vi "Charact One Point.vi"(0 "SG Path in":refnum<class "SG 18GHz Path.lvclass">, 5 "Cal point in":T1, 11 "error in (no error)":errorcluster) -> (4 "SG Path out":refnum<class "SG 18GHz Path.lvclass">, 15 "error out":errorcluster)   [LabVIEW 2023, in "RFFixtureCharact.RFPM.lvlib" / "SG 18GHz Path.lvclass"]
uses:
  SG 18GHz Path.lvclass
  Public/Base Classes/Scalar/Scalar Path/Type Definitions/Cal Point.ctl
  Public/Base Classes/Scalar/SG Abstract Path/SG Abstract Path.lvclass
  Public/Base Classes/Scalar/Scalar Path/Scalar Path.lvclass
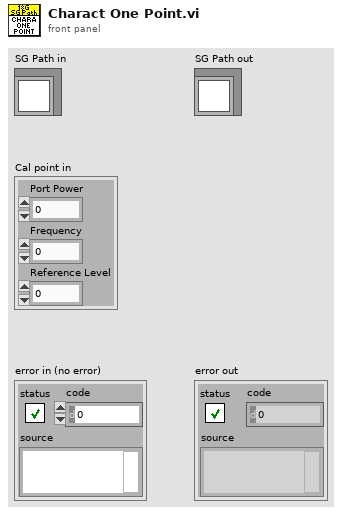
[diagram p1: front panel]
types:
  T1 = typedef "RFFixtureCharact.Public.lvlib/Scalar Path.lvclass/Cal Point.ctl" = cluster{"Port Power":dbl, "Frequency":dbl, "Reference Level":dbl}
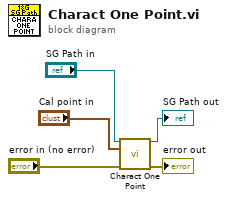
[diagram p0: block diagram]
diagram:
  n1 = call-parent "Charact One Point.vi"("SG Path in"="SG Path in", "Cal point in"="Cal point in", "error in (no error)"="error in (no error)") -> ("SG Path out"=→"SG Path out":refnum<class "SG 18GHz Path.lvclass">, "error out"=→"error out":errorcluster)  [unwired: 11 in]
